vi "p10y1.vi"() -> ()   [LabVIEW 2020]
uses:
  <vilib>/express/express analysis/Spectral/Block/exnSpectralBlock spectral measurements peak poly.vi
  <vilib>/express/express analysis/Spectral/Block/exnSpectralBlock spectral measurements peak array WFM.vi
  <vilib>/express/express analysis/Spectral/XNode/ExpressSpectralMeasurementsBlockNode.xnode
panel:
  out "TAVALINE":waveform(dbl)[](graph)
  out "BAND":dynamicdata(graph)
  out "HIGH":dynamicdata(graph)
  out "LOW":dynamicdata(graph)
  out "Waveform Graph":cluster{"f0":dbl, "df":dbl, "magnitude":dbl[]}[](graph)
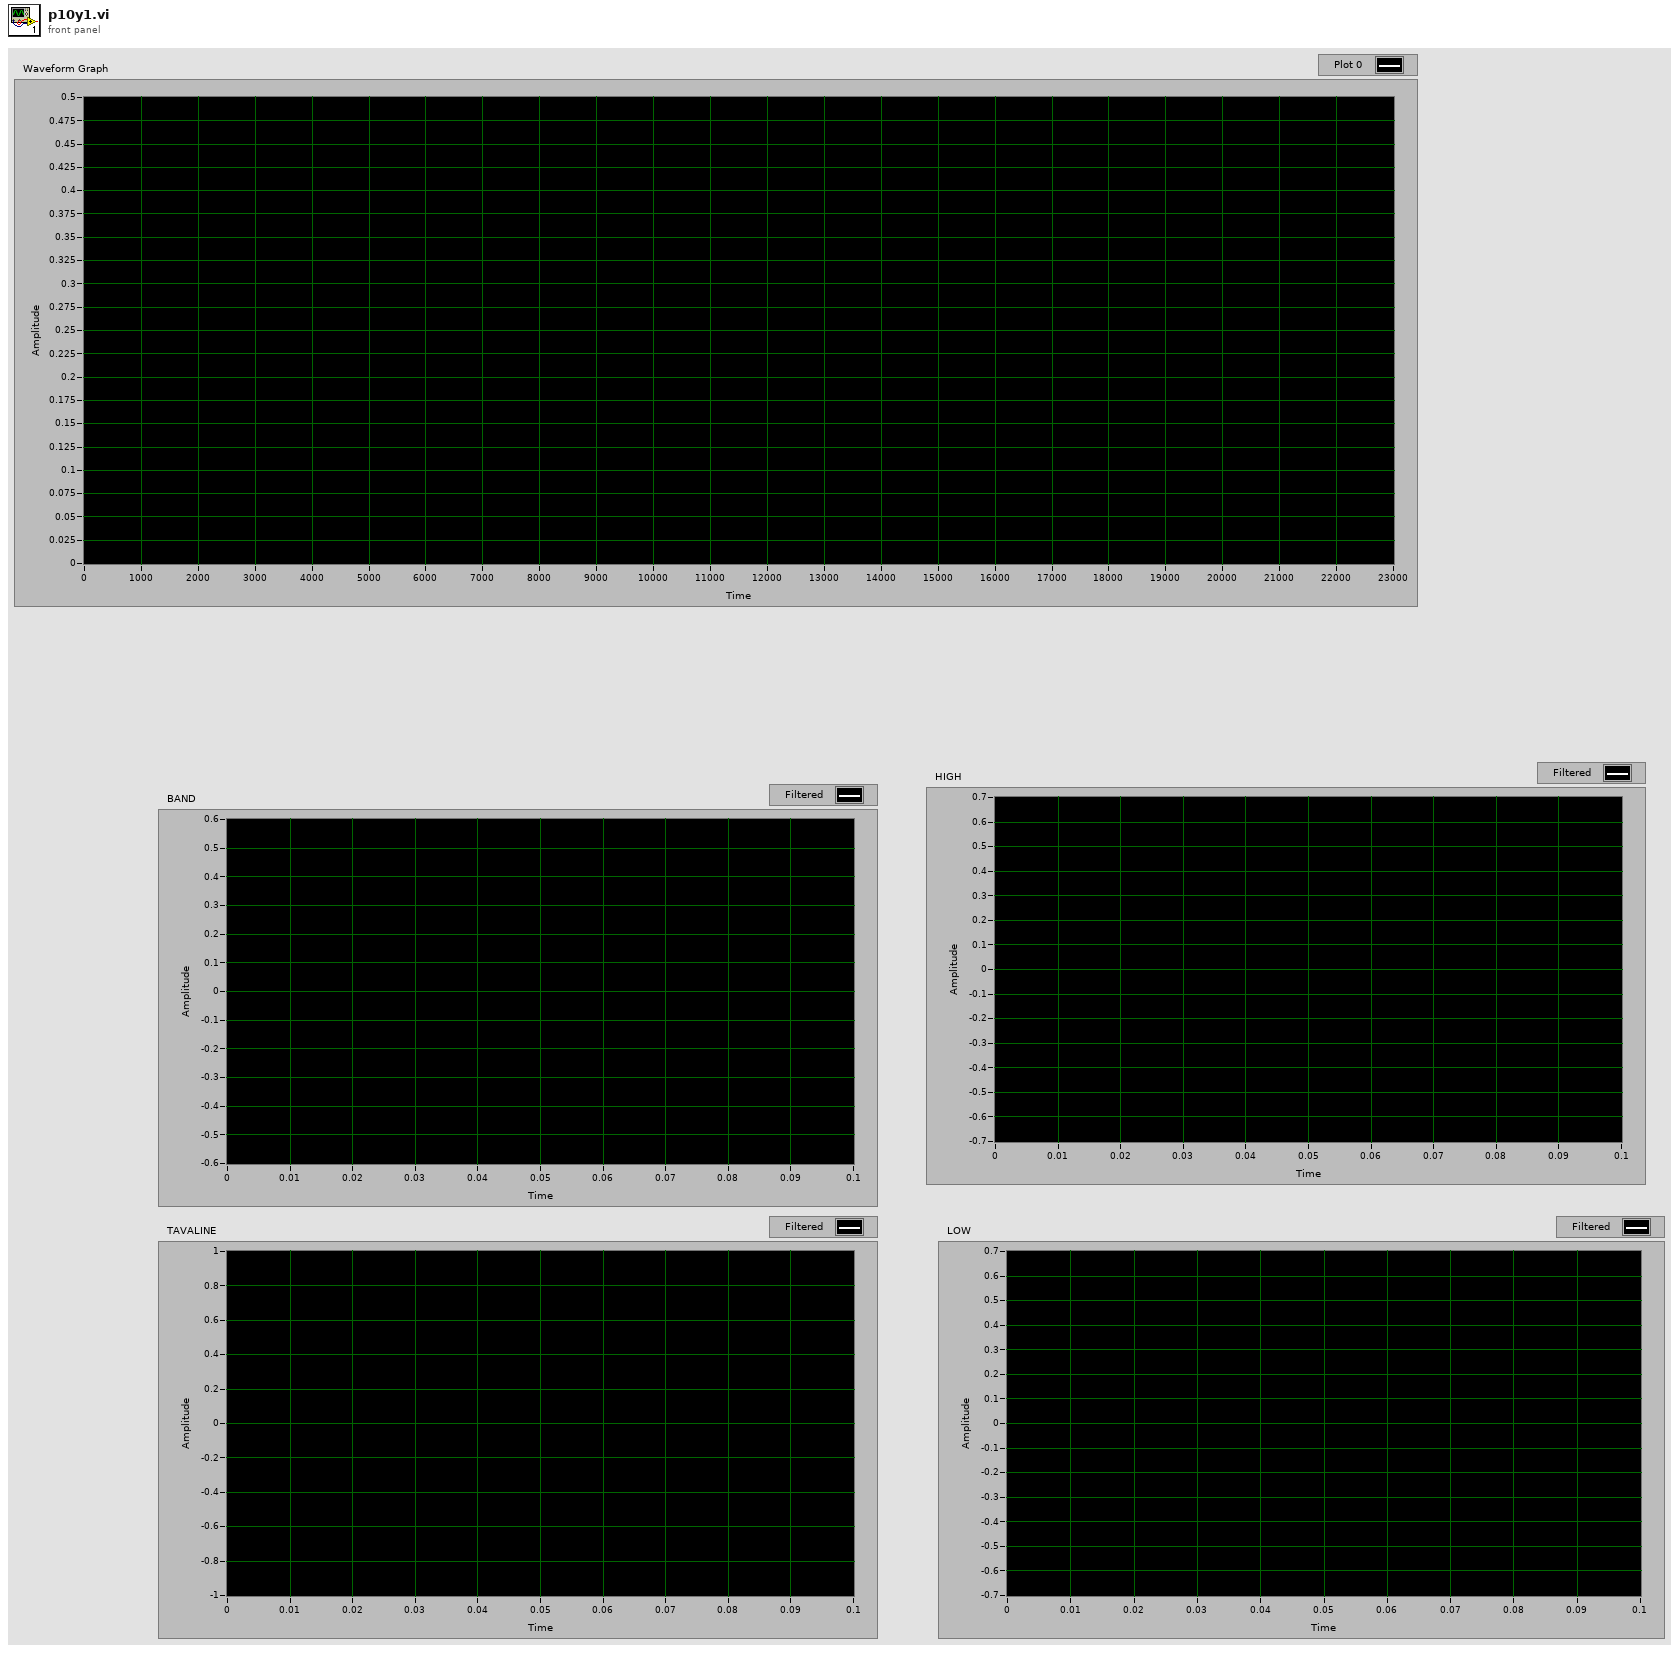
[diagram p1: front panel]
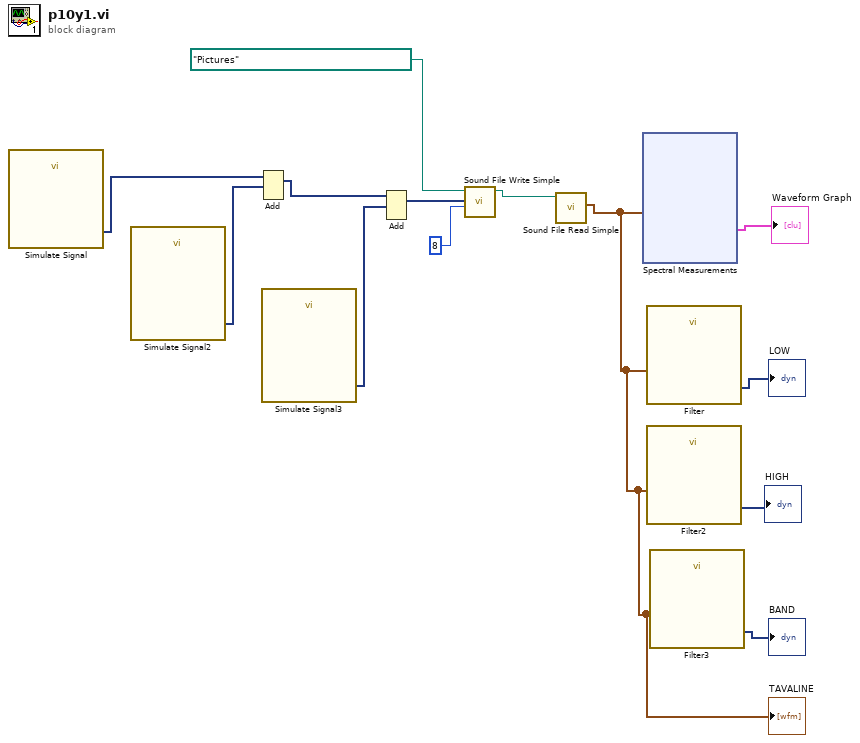
[diagram p0: block diagram]
diagram:
  n1 = call "Simulate Signal"() -> ("Sine"=w13:dynamicdata)  [unwired: 14 in, 1 out]
  n2 = call "Simulate Signal2"() -> ("Sine"=w12:dynamicdata)  [unwired: 14 in, 1 out]
  n3 = Add(1:w12, 2:w13) -> (0:w11:dynamicdata)  [unwired: 1 in, 1 out]
  n4 = call "Simulate Signal3"() -> ("Sine"=w10:dynamicdata)  [unwired: 14 in, 1 out]
  n5 = Add(1:w10, 2:w11) -> (0:w8:dynamicdata)  [unwired: 1 in, 1 out]
  n6 = call <vilib>:"Sound File Write Simple.vi"("bits per sample"=8, "data"=w8, "path"=path "Pictures") -> ("path out"=w6:path)  [unwired: 7 in, 1 out]
  n7 = call <vilib>:"Sound File Read Simple.vi"("path"=w6) -> ("data"=w1:waveform(dbl)[])  [unwired: 7 in, 3 out]
  "TAVALINE" <- w1
  n8 = xnode "Spectral Measurements"("Signals"=w1) -> ("FFT - (Peak)"=→"Waveform Graph":cluster{"f0":dbl, "df":dbl, "magnitude":dbl[]}[])  [unwired: 1 in, 2 out]
  n9 = call "Filter"("Signal"=w1) -> ("Filtered Signal"=→"LOW":dynamicdata)  [unwired: 9 in, 1 out]
  n10 = call "Filter2"("Signal"=w1) -> ("Filtered Signal"=→"HIGH":dynamicdata)  [unwired: 9 in, 1 out]
  n11 = call "Filter3"("Signal"=w1) -> ("Filtered Signal"=→"BAND":dynamicdata)  [unwired: 9 in, 1 out]
